vi "DialogRenameVI.vi"(0 "LibWriter":refnum<class "LibWriter.lvclass">, 1 "VIItemRefIn":refnum<vi>, 5 "error in (no error)":errorcluster) -> (14 "LibWriter":refnum<class "LibWriter.lvclass">, 15 "Cancelled":bool, 16 "RenameOption":T1, 19 "error out":errorcluster)   [LabVIEW 2014, in "LibWriter.lvclass"]
uses:
  <resource>/Framework/Providers/Open_GDS/ClassProviders/LibProvider_BaseClassInterface/LibWriter_class/ClassWriter_class/LibWriter.lvclass
  <resource>/Framework/Providers/Open_GDS/ClassProviders/LibProvider_BaseClassInterface/LibWriter_class/ClassWriter_class/RenameViOption.ctl
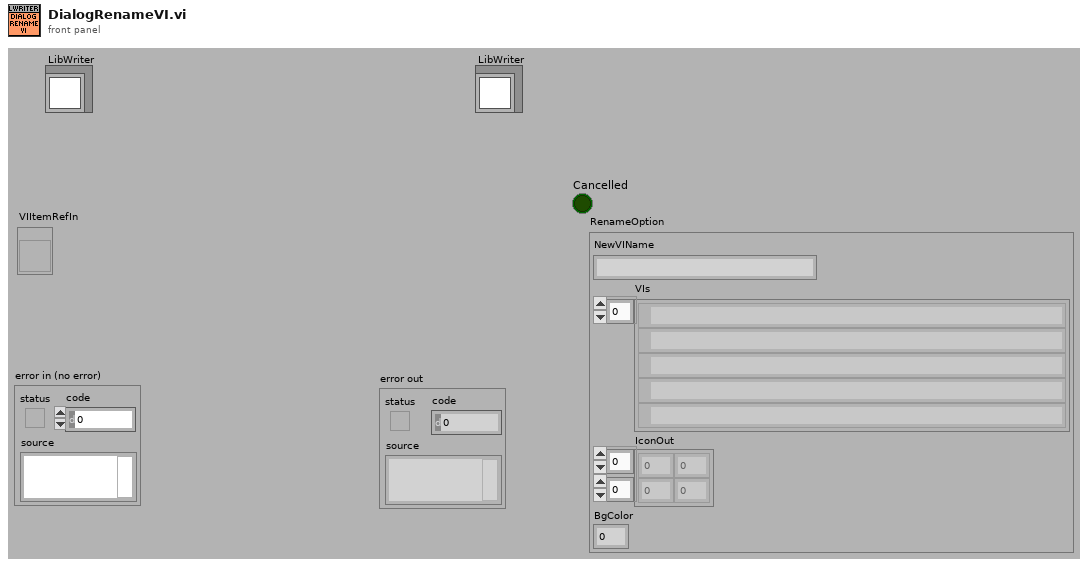
[diagram p1: front panel]
types:
  T1 = typedef "LibWriter.lvclass/RenameViOption.ctl" = cluster{"NewVIName":string, "VIs":path[], "IconOut":u8[][], "BgColor":u8}
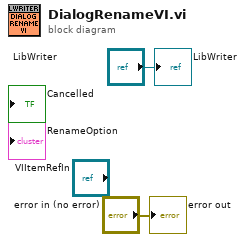
[diagram p0: block diagram]
diagram:
  "error out" <- "error in (no error)"
  "LibWriter" <- "LibWriter"
